vi "RT.vi"() -> ()   [LabVIEW 2015]
uses:
  <vilib>/FPGAPlugInAG/sbRIO-9637/niLvFpga_Open_sbRIO-9637.vi
  <vilib>/rvi/interface/common/dynamic/niFpgaDynamicAddResources.vi
  <vilib>/Utility/error.llb/Error Cluster From Error Code.vi
  <vilib>/rvi/errors/niLvFpgaAdjustHostInterfaceError.vi
  <vilib>/FPGAPlugInAG/Dynamic/niLvFpga_Close_Dynamic.vi
  <vilib>/rvi/interface/nirviOpenFPGA/nirviOpenFPGA.xnode
  FPGA Bitfiles/RIOSPI_FPGATarget_FPGA_Zfin8ch4Lng.lvbitx
  FPGA.vi
  <vilib>/rvi/interface/nirviReadWriteControl/nirviReadWriteControl.xnode
  <vilib>/rvi/interface/nirviCloseFPGA/nirviCloseFPGA.xnode
  NiFpgaLv.dll
  <vilib>/rvi/interface/Simulation/niFpgaSimulationCallBeginRW.vi
panel:
  out "Monitor":u16
  in  "Data":u32(slide) scale=0.0..250.0
  in  "SPI":bool
  out "Error Out":errorcluster
  in  "Error In":errorcluster
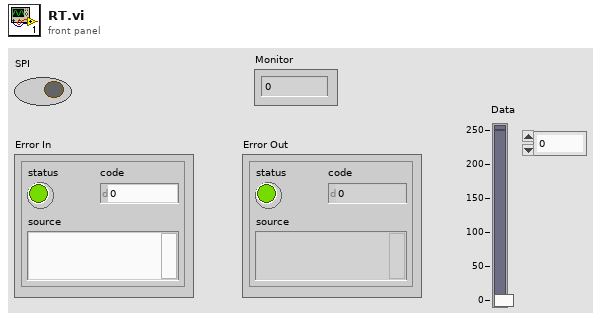
[diagram p1: front panel]
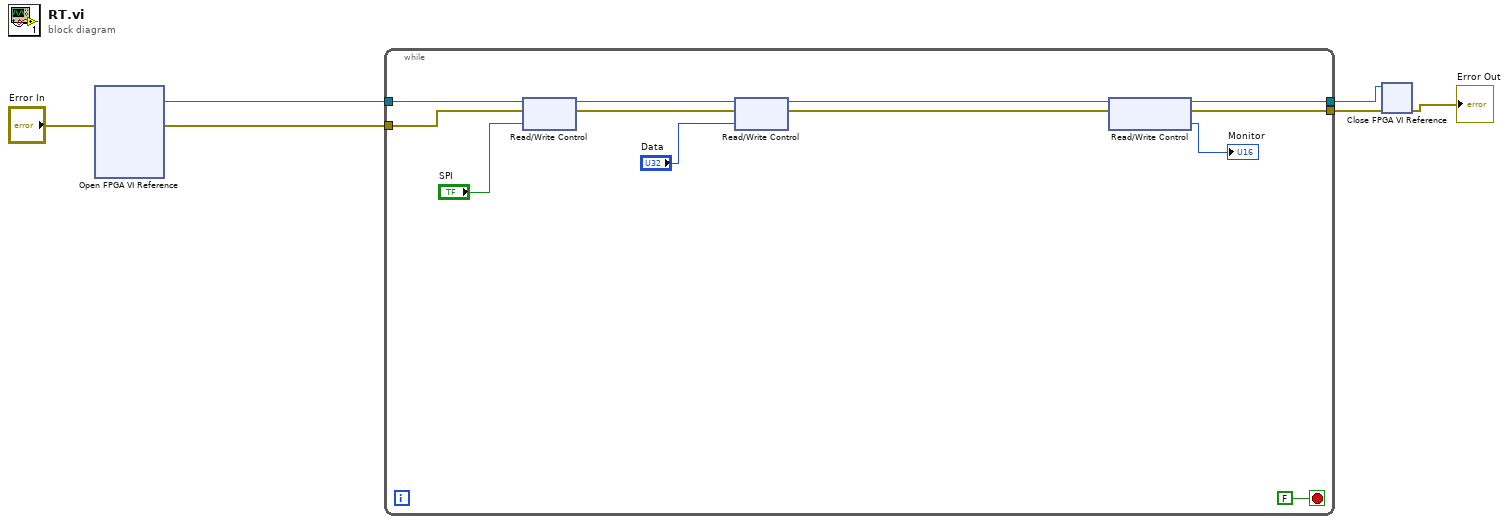
[diagram p0: block diagram]
diagram:
  n1 = xnode "Open FPGA VI Reference"("error in"="Error In") -> ("FPGA VI Reference Out"=w6:refnum<k20>, "error out"=w5:errorcluster)  [unwired: 1 in]
  n2 = while {
    tunnel: w6 -> [w17]
    tunnel: w5 -> [w16]
    tunnel: [w12] -> w2
    tunnel: [w7] -> w1
    stop <- FALSE stop-if-true
    n3 = xnode "Read/Write Control"("FPGA VI Reference In"=w17, "error in"=w16, "Write"="SPI") -> ("FPGA VI Reference Out"=w11:refnum<k20>, "error out"=w14:errorcluster)
    n4 = xnode "Read/Write Control"("FPGA VI Reference In"=w11, "error in"=w14, "Data"="Data") -> ("FPGA VI Reference Out"=w10:refnum<k20>, "error out"=w13:errorcluster)
    n5 = xnode "Read/Write Control"("FPGA VI Reference In"=w10, "error in"=w13) -> ("FPGA VI Reference Out"=w7:refnum<k20>, "error out"=w12:errorcluster, "PIC Monitor"=→"Monitor":u16)
  }
  n6 = xnode "Close FPGA VI Reference"("FPGA VI Reference In"=w1, "error in"=w2) -> ("error out"=→"Error Out":errorcluster)
